vi "SerializeSliceCalcString.vi"(8 "error in (no error)":errorcluster, 10 "Class NameVer":T1[](array[typedef]), 11 "Slice-To-This Class Name":string) -> (0 "error out":errorcluster, 3 "Class":T3[](array[typedef]))   [LabVIEW 2020, in "BlueSerialization.lvlib" / "BlueSerializer.lvclass"]
uses:
  BlueSerializer.lvclass
  Support/GetSerializableDataClusterClass.ctl
  Support/SerializableDataGetDataAction.ctl
  ClassNameAndVersion.ctl
  <vilib>/Utility/EditLVLibs/LibVersion.ctl
  <vilib>/Utility/error.llb/Error Cluster From Error Code.vi
  <vilib>/ErrorRing/Error Ring.xnode
  <vilib>/Utility/EditLVLibs/Edit LVLibs.lvlib
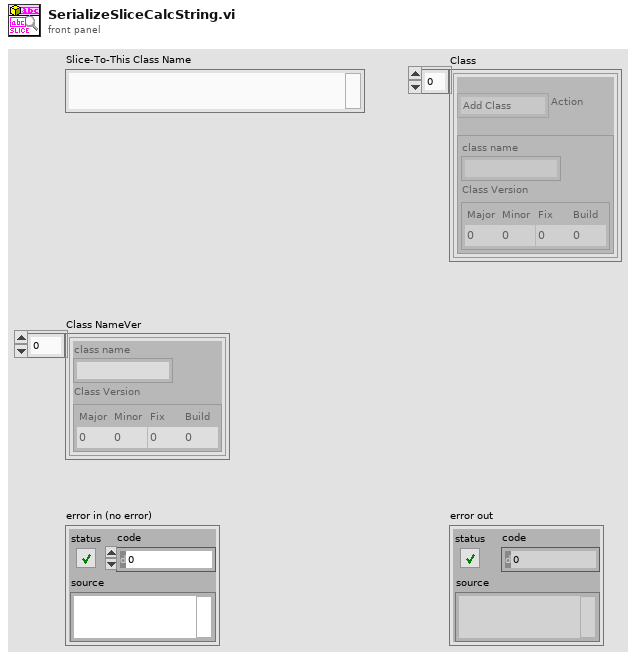
[diagram p1: front panel]
types:
  T1 = typedef "BlueSerialization.lvlib/BlueSerializer.lvclass/ClassNameAndVersion.ctl" = cluster{"class name":string, "Class Version":T2}
  T2 = typedef "Edit LVLibs.lvlib/LibVersion.ctl" = cluster{"Major":u16, "Minor":u16, "Fix":u16, "Build":u16}
  T3 = typedef "BlueSerialization.lvlib/BlueSerializer.lvclass/GetSerializableDataClusterClass.ctl" = cluster{"Action":T4, "Class":T1}
  T4 = typedef "BlueSerialization.lvlib/BlueSerializer.lvclass/SerializableDataGetDataAction.ctl" = enum16{"Add Class", "Drop Class"}
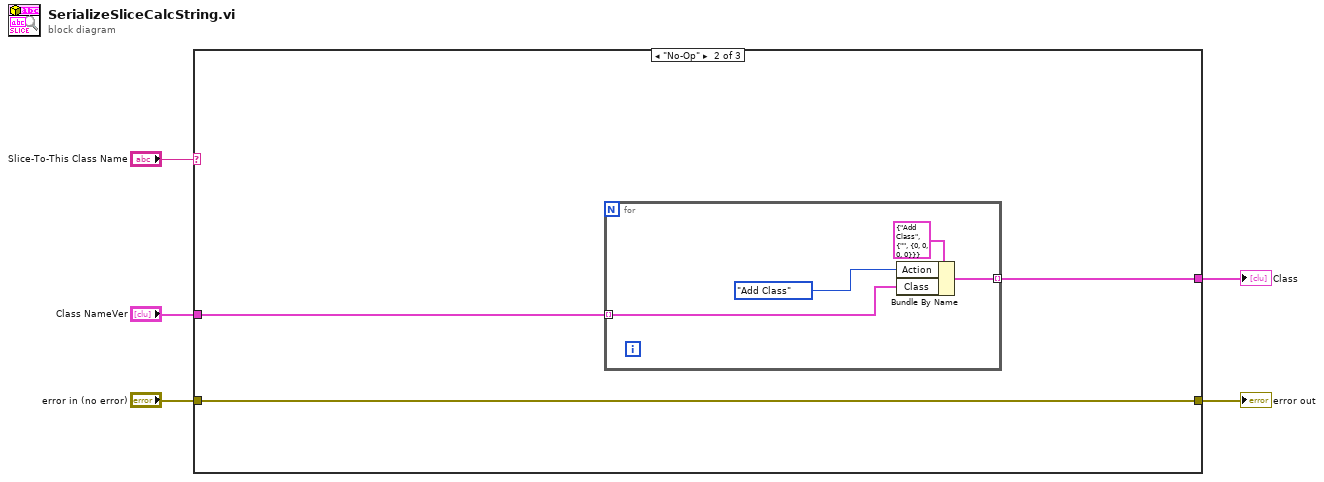
[diagram p0: block diagram]
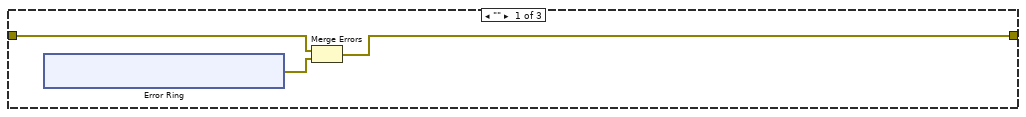
[diagram p2: hidden frame]
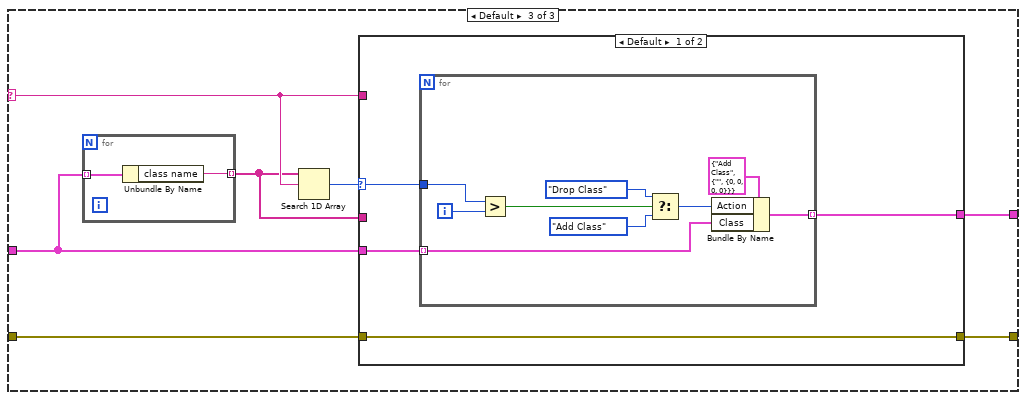
[diagram p3: hidden frame]
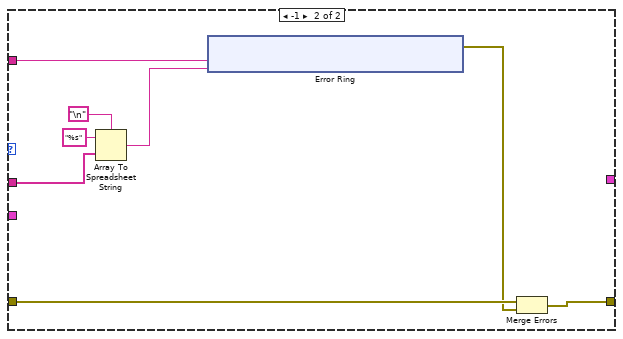
[diagram p4: hidden frame]
diagram:
  n1 = case shown="\"No-Op\"" "Slice-To-This Class Name" {
    selector: "Slice-To-This Class Name" -> [_ _ w24]
    tunnel: [_ w14 w27] -> w5
    tunnel: [w6 w16 w26] -> w4
    tunnel: "error in (no error)" -> [w8 w16 w23]
    tunnel: "Class NameVer" -> [_ w15 w22]
    frame "" {
      n2 = xnode "Error Ring"() -> ("error out"=w7:errorcluster)
      n3 = Merge Errors(w8, w7) -> (w6:errorcluster)
    }
    frame "No-Op" {
      n4 = for {
        tunnel: w15 -> [w18] mode=indexing
        tunnel: [w19] -> w14 mode=indexing
        n5 = Bundle By Name(cluster=T3 {"Action"=enum."Add Class", "Class"={"class name"="", "Class Version"={"Major"=0, "Minor"=0, "Fix"=0, "Build"=0}}} ("Cluster 2"), "Action"=SerializableDataGetDataAction."Add Class", "Class"=w18) -> (w19:T3)
      }
    }
    frame Default {
      n6 = for {
        tunnel: w22 -> [w29] mode=indexing
        tunnel: [w28] -> w21 mode=indexing
        n7 = Unbundle By Name(w29) -> ("class name"=w28:string)
      }
      n8 = Search 1D Array(1D array=w21, element=w24) -> (index of element=w25:i32)  [unwired: 1 in]
      n9 = case shown="Default" w25 {
        selector: w25 -> [w30 _]
        tunnel: w24 -> [_ w50]
        tunnel: w22 -> [w32 _]
        tunnel: w23 -> [w33 w46]
        tunnel: [w33 w44] -> w26
        tunnel: [w31 _] -> w27
        tunnel: w21 -> [_ w43]
        frame Default {
          n10 = for {
            tunnel: w32 -> [w34] mode=indexing
            tunnel: [w41] -> w31 mode=indexing
            tunnel: w30 -> [w40]
            i -> [w39]
            n11 = Greater?(x=w40, y=w39) -> (0:w35:bool)
            n12 = Select(t=SerializableDataGetDataAction."Drop Class" ("Action"), s=w35, f=SerializableDataGetDataAction."Add Class" ("Action")) -> (s? t:f=w36:T4)
            n13 = Bundle By Name(cluster=T3 {"Action"=enum."Add Class", "Class"={"class name"="", "Class Version"={"Major"=0, "Minor"=0, "Fix"=0, "Build"=0}}} ("Cluster 2"), "Action"=w36, "Class"=w34) -> (w41:T3)
          }
        }
        frame -1 {
          n14 = Array To Spreadsheet String(delimiter (Tab)="\n", array=w43, 3:"%s" ("format string")) -> (spreadsheet string=w47:string)
          n15 = xnode "Error Ring"("parameter 0"=w50, "parameter 1"=w47) -> ("error out"=w45:errorcluster)
          n16 = Merge Errors(w46, w45) -> (w44:errorcluster)
        }
      }
    }
  }
  "Class" <- w5
  "error out" <- w4
